vi "array -- smart enum -- test.vi"() -> ()   [LabVIEW 2012]
uses:
  hash action control.ctl
panel:
  out "hash key OUT":string
  out "index OUT":i32
  out "found?":bool
  in  "index IN":i32
  in  "hash key":string
  in  "hash action":T1
  in  "angle":u16(ring) items=["", "-9"]
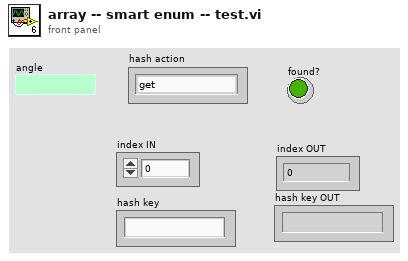
[diagram p1: front panel]
types:
  T1 = typedef "hash action control.ctl" = enum16{"get", "new", "--void", "delete", "delete all", "set", "--delete if exists", "--create if not there", "list keys", "index forw", "index back", "check", "index set"}
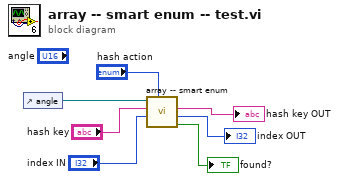
[diagram p0: block diagram]
diagram:
  n1 = control-ref of="angle"() -> (w6:refnum<vi>)
  n2 = call "array -- smart enum.vi"("hash action"="hash action", "index IN"="index IN", "hash key"="hash key", "hash"=w6) -> ("found?"=→"found?":bool, "index OUT"=→"index OUT":i32, "hash key OUT"=→"hash key OUT":string)  [unwired: 3 in, 2 out]
